vi "Untitled 1.vi"() -> ()   [LabVIEW 2018]
uses:
  RRT.dll
panel:
  out "NT":dbl[](array[numeric])
  out "return type":i32
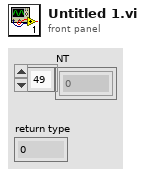
[diagram p1: front panel]
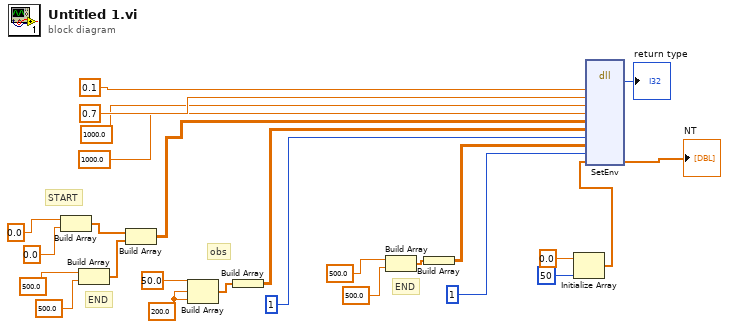
[diagram p0: block diagram]
diagram:
  w14 = 200.0
  # "END"
  # "obs"
  # "END"
  # "START"
  n1 = Build Array(0.0, 0.0) -> (w18:dbl[])
  n2 = Build Array(500.0, 500.0) -> (w17:dbl[])
  n3 = Build Array(w18, w17) -> (w16:dbl[][])
  n4 = Build Array(50.0, w14, w14) -> (w13:dbl[])
  n5 = Build Array(w13) -> (w12:dbl[][])
  n6 = Build Array(500.0, 500.0) -> (w8:dbl[])
  n7 = Build Array(w8) -> (w7:dbl[][])
  n8 = Initialize Array(0.0, 50) -> (w3:dbl[])
  n9 = dll-call lib="C:/Users/anton/source/repos/RRT/x64/Release/RRT.dll" fn="SetEnv"("pgoal"=0.1, "pway"=0.7, "fl"=1000.0, "fw"=1000.0, "se"=w16, "o"=w12, "ol"=1, "lt"=w7, "ltL"=1, "NT"=w3) -> ("return type"=→"return type":i32, "NT"=→"NT":dbl[])  [unwired: 12 in, 2 out]
